vi "Tag Text.vi"(3 "Value":string, 4 "properties":string, 5 "Tag":string) -> (1 "tagged string":string)   [LabVIEW 2020, in "XmlInterface.lvclass"]
uses:
  XmlInterface.lvclass
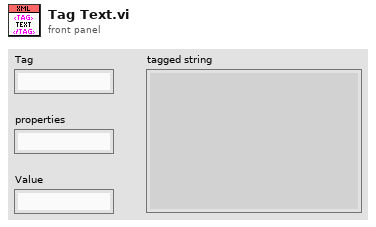
[diagram p1: front panel]
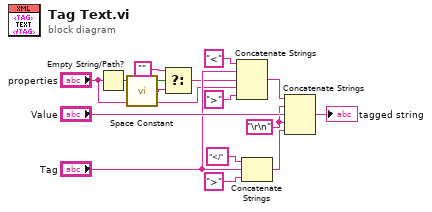
[diagram p0: block diagram]
diagram:
  w6 = "\r\n"
  n1 = Empty String/Path?(string/path="properties") -> (empty?=w4:bool)
  n2 = call <vilib>:"Space Constant.vi"() -> ("String"=w3:string)
  n3 = Select(t="", s=w4, f=w3) -> (s? t:f=w1:string)
  n4 = Concatenate Strings("<" ("string"), "Tag", w1, "properties", ">" ("string")) -> (w11:string)
  n5 = Concatenate Strings("</" ("string"), "Tag", ">" ("string")) -> (w9:string)
  n6 = Concatenate Strings(w11, w6, "Value", w6, w9) -> (→"tagged string":string)
